vi "ControlMainGUIWindow.vi"(8 "Error In":errorcluster, 10 "ShowProcessWindow":bool, 11 "reference in":refnum<class "UserManager.lvclass">) -> (0 "Error Out":errorcluster, 2 "Dummy":bool, 3 "reference out":refnum<class "UserManager.lvclass">)   [LabVIEW 2021, in "UserMananger.lvlib" / "UserManager.lvclass"]
uses:
  UserManager.lvclass
  protected/UserManager_MessageData.ctl
  9f903c85-2847-4db9-ba05-d8e85b2316fc.vi
  protected/MainGUIRepository.vi
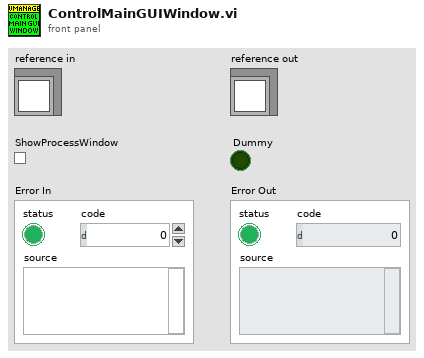
[diagram p1: front panel]
types:
  T1 = typedef "UserMananger.lvlib/UserManager.lvclass/UserManager_MessageData.ctl" = cluster{"ShowWindow":cluster{"Send":cluster{"Show":bool}, "Receive":cluster{"Dummy":bool}}}
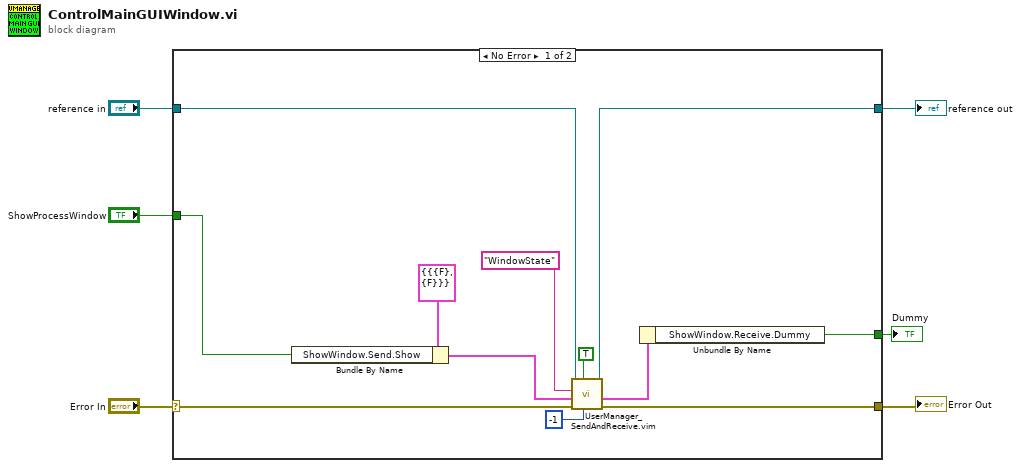
[diagram p0: block diagram]
diagram:
  n1 = case shown="No Error" "Error In" {
    selector: "Error In" -> [w18 w20]
    tunnel: [w17 w20] -> w5
    tunnel: [w14 w19] -> w3
    tunnel: "reference in" -> [w15 w19]
    tunnel: "ShowProcessWindow" -> [w12 _]
    tunnel: [w9 _] -> w1
    frame No Error {
      n2 = Bundle By Name(cluster=T1 {"ShowWindow"={"Send"={"Show"=FALSE}, "Receive"={"Dummy"=FALSE}}} ("MessageData"), "ShowWindow.Send.Show"=w12) -> (w11:T1)
      n3 = call "UserManager_SendAndReceive.vim"("timeout in ms (-1)"=-1, "ShouldWeWaitForResponse"=TRUE, "error in (no error)"=w18, "Data"=w11, "Command"="WindowState", "reference in"=w15) -> ("error out"=w17:errorcluster, "ReplyData"=w10:T1, "reference out"=w14:refnum<class "UserManager.lvclass">)  [unwired: 3 in]
      n4 = Unbundle By Name(w10) -> ("ShowWindow.Receive.Dummy"=w9:bool)
    }
    frame Error {
    }
  }
  "Error Out" <- w5
  "reference out" <- w3
  "Dummy" <- w1
